vi "Light Sensor Array.vi"(2 "NXT":T2={"Hardware"="NXT", "Flattened String"=""}, 3 "Input Port":T1 items=["Port 1", "Port 2", "Port 3", "Port 4"]) -> (1 "output cluster":cluster{u8, u8, u8, u8, u8, u8, u8, u8}, 4 "NXT dup":T2={"Hardware"="NXT", "Flattened String"=""} caption="NXT")   [LabVIEW 2010]
uses:
  <vilib>/NXT/Subs/LVHSConnector.ctl
  <vilib>/NXT/Block Support/NXT_InputPort.ctl
  <vilib>/NXT/Block Support/HWPage.SensorType.ctl
  <vilib>/NXT/Block Support/HWPage.SensorMode.ctl
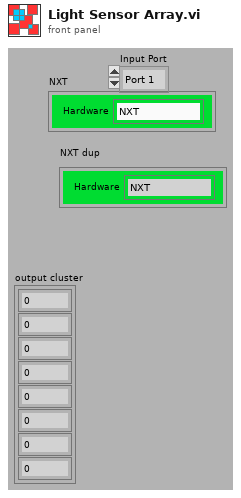
[diagram p1: front panel]
types:
  T1 = typedef "NXT_InputPort.ctl" = u8
  T2 = typedef "LVHSConnector.ctl" = cluster{"Hardware":string, "Flattened String":string}
  T3 = typedef "HWPage.SensorType.ctl" = u8
  T4 = typedef "HWPage.SensorMode.ctl" = u8
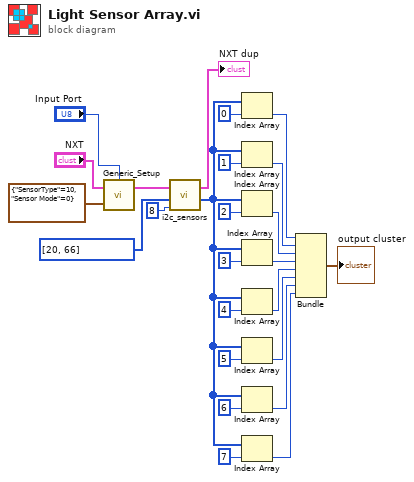
[diagram p0: block diagram]
diagram:
  n1 = call <vilib>:"Generic_Setup.vi"("Sensor Setup"=cluster{"SensorType":T3, "Sensor Mode":T4} {"SensorType"=10, "Sensor Mode"=0}, "NXT"="NXT", "Port"="Input Port") -> ("NXT"=w22:T2)  [unwired: 1 out]
  n2 = call <vilib>:"i2c_sensors.vi"("Return Length"=u8 8, "Bytes to Write"=u8[] [20, 66], "NXT"=w22) -> ("Bytes read"=w11:u8[], "NXT"=→"NXT dup":T2)  [unwired: 2 in, 1 out]
  n3 = Index Array(array=w11, index=0) -> (element=w10:u8)
  n4 = Index Array(array=w11, index=1) -> (element=w9:u8)
  n5 = Index Array(array=w11, index=2) -> (element=w8:u8)
  n6 = Index Array(array=w11, index=3) -> (element=w7:u8)
  n7 = Index Array(array=w11, index=4) -> (element=w6:u8)
  n8 = Index Array(array=w11, index=5) -> (element=w5:u8)
  n9 = Index Array(array=w11, index=6) -> (element=w4:u8)
  n10 = Index Array(array=w11, index=7) -> (element=w3:u8)
  n11 = Bundle(w10, w9, w8, w7, w6, w5, w4, w3) -> (→"output cluster":cluster{u8, u8, u8, u8, u8, u8, u8, u8})  [unwired: 1 in]
